vi "Drive-Rotate-Camera_Track.vi"(0 "Ball X":dbl, 1 "Valid Ball?":bool, 2 "Desired Distance":dbl format="%.2f", 3 "Left Encoder":dbl, 4 "Right Encoder":dbl, 5 "Drive Mode":T3(ring), 7 "Controller X":dbl, 9 "Controller Y":dbl, 11 "Controller Rotate":dbl, 13 "Strafe?":bool, 16 "Ball X Time":dbl, 17 "Eval Period (sec)":dbl(knob)=0.1607904282898374 scale=0.0..1.0, 18 "Gyro Angle":dbl, 19 "Desired Angle":dbl) -> (6 "Rotate Out":dbl, 8 "X Out":dbl, 10 "Y Out":dbl, 12 "Stable":bool, 14 "F Mode":bool, 15 "Filtered":dbl)   [LabVIEW 2013]
uses:
  <vilib>/addons/control/pid/pid.llb/PID (DBL).vi
  <vilib>/addons/control/pid/NI_PID_pid.lvlib
panel:
  in  "Tab Control":T1(tab)
  in  "Drive Forward":dbl=0.8
  in  "Rate Thresh":dbl=600.0 step=0.001
  in  "Rotate Tol":dbl=0.75
  in  "Stop Rotate PID":T2={"proportional gain (Kc)"=0.03, "integral time (Ti, min)"=0.01, "derivative time (Td, min)"=0.003} {"derivative time (Td, min)" format="%.3f"; "integral time (Ti, min)" format="%.3f"; "proportional gain (Kc)" format="%.3f"}
  in  "Track PID":T2={"proportional gain (Kc)"=0.09, "integral time (Ti, min)"=0.003, "derivative time (Td, min)"=0.001} {"derivative time (Td, min)" format="%.3f"; "integral time (Ti, min)" format="%.3f"; "proportional gain (Kc)" format="%.3f"}
  in  "Rotate PID":T2={"proportional gain (Kc)"=0.04, "integral time (Ti, min)"=0.01, "derivative time (Td, min)"=0.001} {"derivative time (Td, min)" format="%.3f"; "integral time (Ti, min)" format="%.3f"; "proportional gain (Kc)" format="%.3f"}
  # "Left side is input\nRight side is within VI control"
  # "12 in\n4 out"
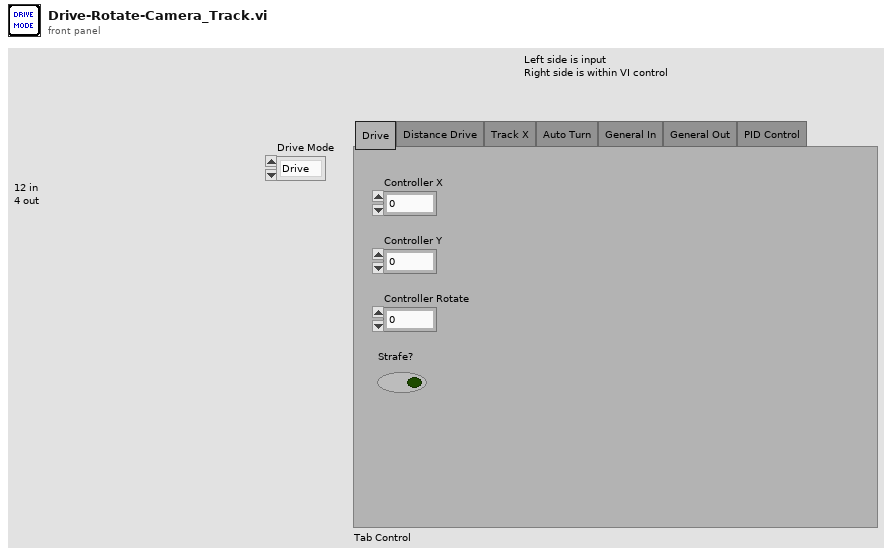
[diagram p1: front panel]
types:
  T1 = enum32{"Drive", "Distance Drive", "Track X", "Auto Turn", "General In", "General Out", "PID Control"}
  T2 = cluster{"proportional gain (Kc)":dbl, "integral time (Ti, min)":dbl, "derivative time (Td, min)":dbl}
  T3 = enum16{"Drive", "Rotate", "Track X", "Distance Drive"}
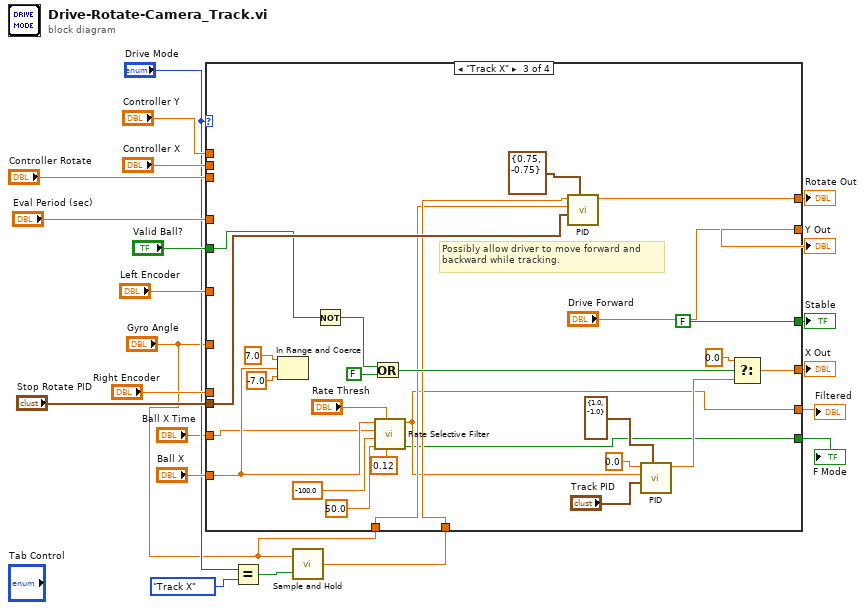
[diagram p0: block diagram]
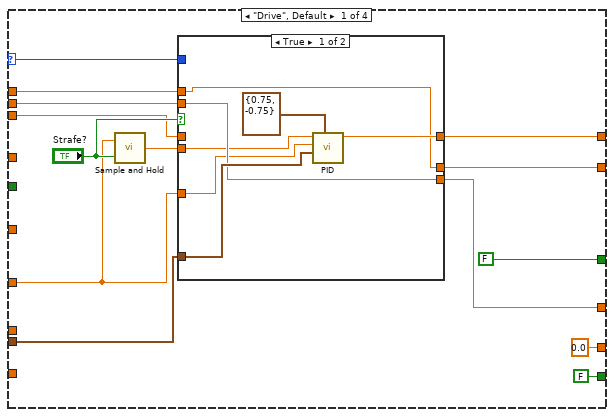
[diagram p2: hidden frame]
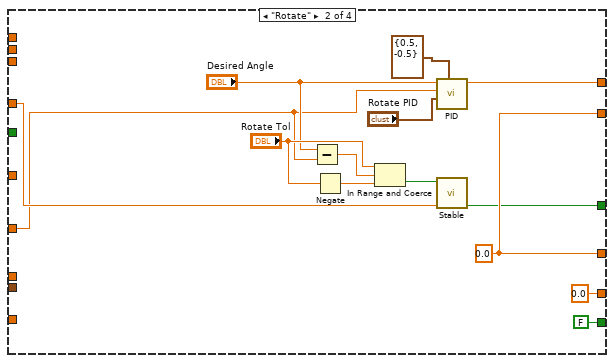
[diagram p4: hidden frame]
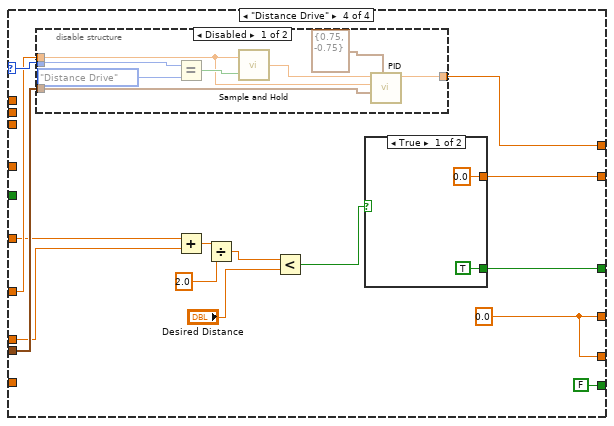
[diagram p5: hidden frame]
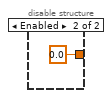
[diagram p6: hidden frame]
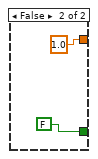
[diagram p7: hidden frame]
diagram:
  n1 = Equal?(x="Drive Mode", y=enum16{"Drive", "Rotate", "Track X"}."Track X") -> (x = y?=w8:bool)
  n2 = call "Sample and Hold.vi"("Hold?"=w8, "Input"="Gyro Angle") -> ("Output"=w5:dbl)
  n3 = case shown="\"Track X\"" "Drive Mode" {
    selector: "Drive Mode" -> [w29 _ _ w101]
    tunnel: [w33 w58 w77 w99] -> w21
    tunnel: [w31 w57 w69 w88] -> w20
    tunnel: [w32 w57 "Drive Forward" w93] -> w19
    tunnel: "Controller X" -> [w34 _ _ _]
    tunnel: "Controller Y" -> [w35 _ _ _]
    tunnel: "Controller Rotate" -> [w27 _ _ _]
    tunnel: "Stop Rotate PID" -> [w30 _ w86 w100]
    tunnel: [FALSE ("Stable") w52 FALSE ("Stable") w92] -> w14
    tunnel: "Eval Period (sec)" -> [_ w49 _ _]
    tunnel: "Gyro Angle" -> [w24 w48 _ w98]
    tunnel: "Ball X" -> [_ _ w68 _]
    tunnel: "Valid Ball?" -> [_ _ w73 _]
    tunnel: "Right Encoder" -> [_ _ _ w97]
    tunnel: "Left Encoder" -> [_ _ _ w96]
    tunnel: w5 -> [_ _ w72 _]
    tunnel: "Gyro Angle" -> [_ _ w71 _]
    tunnel: "Ball X Time" -> [_ _ w64 _]
    tunnel: [0.0 ("Filtered") 0.0 ("Filtered") w63 w88] -> w2
    tunnel: [FALSE ("Mode") FALSE ("Mode") w62 FALSE ("Mode")] -> w1
    frame "Drive", Default {
      n4 = call "Sample and Hold.vi"("Hold?"="Strafe?", "Input"=w24) -> ("Output"=w26:dbl)
      n5 = case shown="True" "Strafe?" {
        tunnel: w35 -> [w36 w45]
        tunnel: w34 -> [w39 w44]
        tunnel: [w42 w43] -> w33
        tunnel: [w36 w45] -> w32
        tunnel: [w39 w44] -> w31
        tunnel: w30 -> [w41 _]
        tunnel: w29 -> [_ _]
        tunnel: w27 -> [_ w43]
        tunnel: w26 -> [w38 _]
        tunnel: w24 -> [w37 _]
        frame True {
          n6 = call-poly <vilib>:"PID.vi"("output range"=cluster{"output high":dbl, "output low":dbl} {"output high"=0.75, "output low"=-0.75}, "PID gains"=w41, "process variable"=w37, "setpoint"=w38) -> ("output"=w42:dbl)  [unwired: 6 in, 1 out]
        }
        frame False {
        }
      }
    }
    frame "Rotate" {
      w57 = 0.0
      n7 = Subtract(x="Desired Angle", y=w48) -> (x-y=w56:dbl)
      n8 = Negate(x="Rotate Tol") -> (-x=w55:dbl)
      n9 = In Range and Coerce(upper limit="Rotate Tol", x=w56, lower limit=w55) -> (In Range?=w53:bool)  [unwired: 1 out]
      n10 = call-poly <vilib>:"PID.vi"("output range"=cluster{"output high":dbl, "output low":dbl} {"output high"=0.5, "output low"=-0.5}, "PID gains"="Rotate PID", "process variable"=w48, "setpoint"="Desired Angle") -> ("output"=w58:dbl)  [unwired: 6 in, 1 out]
      n11 = call "Stable.vi"("Eval Period (sec)"=w49, "Signal Input"=w53) -> ("Stable"=w52:bool)  [unwired: 9 in]
    }
    frame "Track X" {
      # "Possibly allow driver to move forward and\nbackward while tracking."
      n12 = In Range and Coerce(upper limit=7.0, x=w68, lower limit=-7.0) -> ()  [unwired: 2 out]
      n13 = Not(x=w73) -> (.not. x?=w74:bool)
      n14 = Or(x=w74, y=FALSE) -> (x .or. y?=w80:bool)
      n15 = call "Rate Selective Filter.vi"("Hyster"=0.12, "Rate Thresh"="Rate Thresh", "hi limit"=50.0, "lo limit"=-100.0, "Time"=w64, "Distance"=w68) -> ("Mode"=w62:bool, "Filtered"=w63:dbl)  [unwired: 1 in, 1 out]
      n16 = call-poly <vilib>:"PID.vi"("output range"=cluster{"output high":dbl, "output low":dbl} {"output high"=0.75, "output low"=-0.75}, "PID gains"=w86, "process variable"=w71, "setpoint"=w72) -> ("output"=w77:dbl)  [unwired: 6 in, 1 out]
      n17 = call-poly <vilib>:"PID.vi"("output range"=cluster{"output high":dbl, "output low":dbl} {"output high"=1.0, "output low"=-1.0}, "PID gains"="Track PID", "process variable"=w63, "setpoint"=0.0) -> ("output"=w79:dbl)  [unwired: 6 in, 1 out]
      n18 = Select(t=0.0, s=w80, f=w79) -> (s? t:f=w69:dbl)
    }
    frame "Distance Drive" {
      w88 = 0.0 ("output")
      n19 = disable-structure shown="Disabled" {
        disable-tunnel: w101 -> [w106 _]
        disable-tunnel: w100 -> [w105 _]
        disable-tunnel: [w104 0.0 ("output")] -> w99
        disable-tunnel: w98 -> [w103 _]
        frame Disabled {
          n20 = Equal?(x=w106, y=T3."Distance Drive" ("Drive Mode")) -> (x = y?=w108:bool)
          n21 = call "Sample and Hold.vi"("Hold?"=w108, "Input"=w103) -> ("Output"=w107:dbl)
          n22 = call-poly <vilib>:"PID.vi"("output range"=cluster{"output high":dbl, "output low":dbl} {"output high"=0.75, "output low"=-0.75}, "PID gains"=w105, "process variable"=w103, "setpoint"=w107) -> ("output"=w104:dbl)  [unwired: 6 in, 1 out]
        }
        frame Enabled {
        }
      }
      n23 = Add(x=w96, y=w97) -> (x+y=w95:dbl)
      n24 = Divide(x=w95, y=2.0) -> (x/y=w90:dbl)
      n25 = Less?(x=w90, y="Desired Distance") -> (x < y?=w91:bool)
      n26 = case shown="True" w91 {
        tunnel: [0.0 1.0] -> w93
        tunnel: [TRUE FALSE] -> w92
        frame True {
        }
        frame False {
        }
      }
    }
  }
  "Rotate Out" <- w21
  "X Out" <- w20
  "Y Out" <- w19
  "Stable" <- w14
  "Filtered" <- w2
  "F Mode" <- w1
